vi "Explorer auto populate folder.vi"(4 "Folders to Exclude":string[](array[string]), 6 "Pattern":string, 8 "error in (no error)":errorcluster, 9 "Continue Recursing on Error? (F)":bool, 10 "Item Indent":i32, 11 "Folder Path":path) -> (0 "error out":errorcluster, 2 "Items":T1(array[cluster]), 3 "dup Folder Path":path)   [LabVIEW 2015]
doc: "Lists content of a folder as tree items and creates a glyph cache based on file extensions. If a file extension is not cached, this appends the default system shell icon.\n\nCreated By: Ryan Pacini"
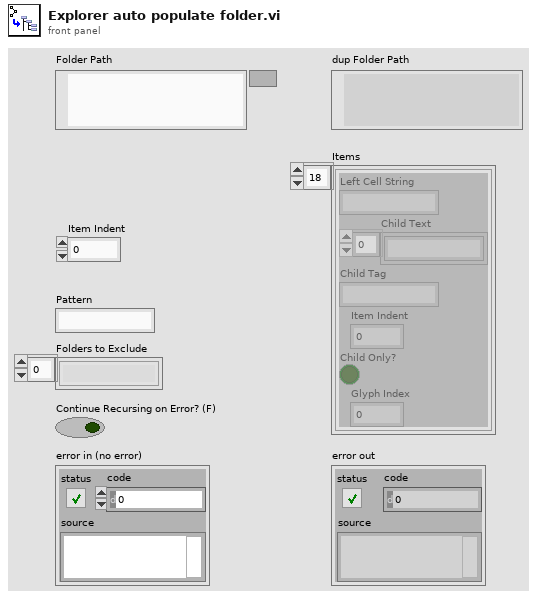
[diagram p1: front panel]
types:
  T1 = cluster{"Left Cell String":string, "Child Text":string[], "Child Tag":string, "Item Indent":i32, "Child Only?":bool, "Glyph Index":i32}[]
  T2 = cluster{"Left Cell String":string, "Child Text":string[], "Child Tag":string, "Item Indent":i32, "Child Only?":bool, "Glyph Index":i32}
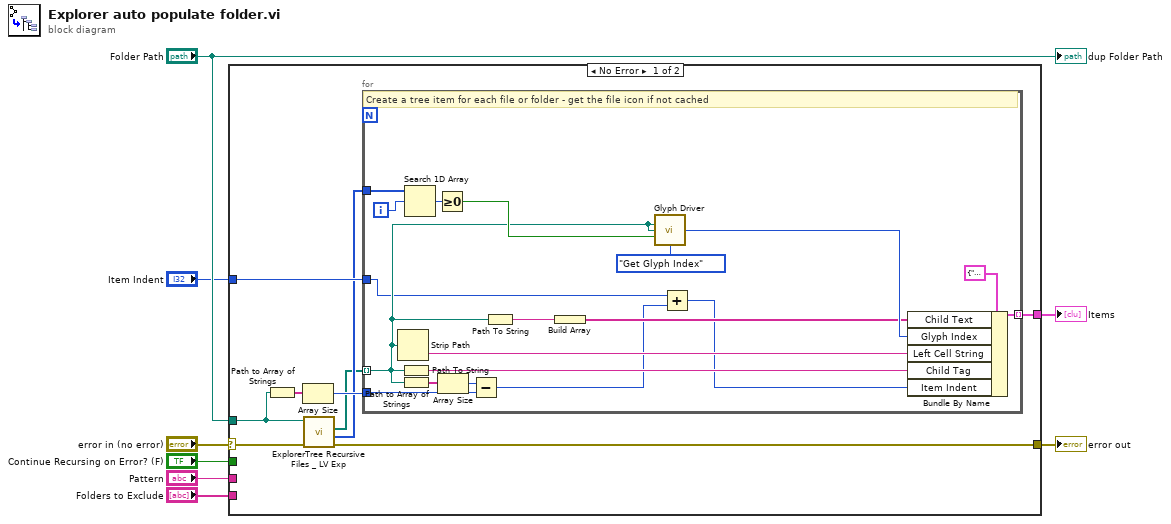
[diagram p0: block diagram]
diagram:
  n1 = case shown="No Error" "error in (no error)" {
    selector: "error in (no error)" -> [w13 w37]
    tunnel: "Pattern" -> [_ _]
    tunnel: [w11 w37] -> w7
    tunnel: "Continue Recursing on Error? (F)" -> [_ _]
    tunnel: "Folder Path" -> [w12 _]
    tunnel: "Folders to Exclude" -> [_ _]
    tunnel: [w15 _] -> w2
    tunnel: "Item Indent" -> [w14 _]
    frame No Error {
      n2 = Path to Array of Strings(0:w12) -> (2:w17:string[])  [unwired: 1 out]
      n3 = Array Size(array=w17) -> (size(s)=w16:i32)
      n4 = call "ExplorerTree Recursive Files _ LV Exp.vi"("error in (no error)"=w13, "Folder Path"=w12) -> ("error out"=w11:errorcluster, "Folder Indexes"=w10:i32[], "Folders and Files"=w9:path[])  [unwired: 6 in, 1 out]
      n5 = for {
        tunnel: w16 -> [w32]
        tunnel: w9 -> [w22] mode=indexing
        tunnel: [w31] -> w15 mode=indexing
        tunnel: w10 -> [w27]
        tunnel: w14 -> [w20]
        i -> [w26]
        # "Create a tree item for each file or folder - get the file icon if not cached"
        n6 = Strip Path(path=w22) -> (name=w30:string)  [unwired: 1 out]
        n7 = Path To String(path=w22) -> (string=w35:string)
        n8 = Path to Array of Strings(0:w22) -> (2:w34:string[])  [unwired: 1 out]
        n9 = Search 1D Array(1D array=w27, element=w26) -> (index of element=w28:i32)  [unwired: 1 in]
        n10 = Greater Or Equal To 0?(x=w28) -> (x >= 0?=w25:bool)
        n11 = Array Size(array=w34) -> (size(s)=w33:i32)
        n12 = Subtract(x=w33, y=w32) -> (x-y=w19:i32)
        n13 = Path To String(path=w22) -> (string=w21:string)
        n14 = Build Array(w21) -> (w23:string[])
        n15 = call "Glyph Driver.vi"("File Path"=w22, "File Relative Path"=w22, "Is Folder?"=w25, "Op Mode"=enum16{"Get Glyph Index", "Get all Glyphs"}."Get Glyph Index") -> ("Glyph Index"=w24:i32)  [unwired: 9 in, 2 out]
        n16 = Add(x=w20, y=w19) -> (x+y=w18:i32)
        n17 = Bundle By Name(cluster=T2 {"Left Cell String"="", "Child Text"=[], "Child Tag"="", "Item Indent"=0, "Child Only?"=FALSE, "Glyph Index"=0} ("Item"), "Child Text"=w23, "Glyph Index"=w24, "Left Cell String"=w30, "Child Tag"=w35, "Item Indent"=w18) -> (w31:T2)
      }
    }
    frame Error {
    }
  }
  "error out" <- w7
  "Items" <- w2
  "dup Folder Path" <- "Folder Path"
